vi "retrieveData.vi"(8 "error in (no error)":errorcluster, 11 "TemperatureSensor in":refnum<class "TemperatureSensor.lvclass">) -> (0 "error out":errorcluster, 2 "Temperature Measured":dbl[unit], 3 "TemperatureSensor out":refnum<class "TemperatureSensor.lvclass">)   [LabVIEW 2013, in "TemperatureSensor.lvclass"]
uses:
  TemperatureSensor.lvclass
  TemperatureSensor.lvclass/TemperatureSensor.ctl
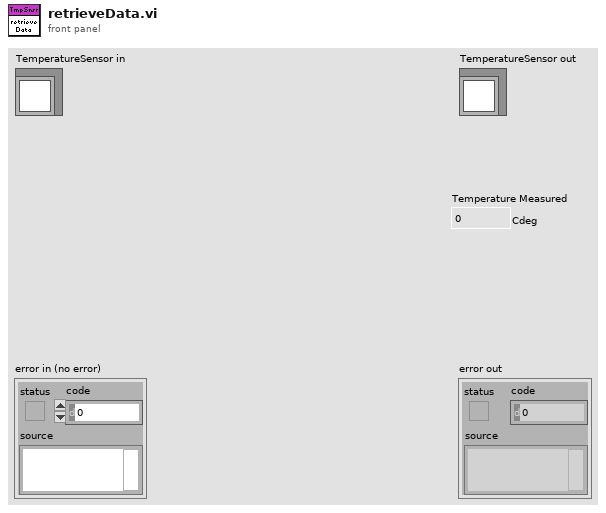
[diagram p1: front panel]
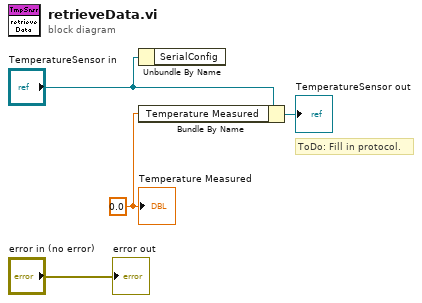
[diagram p0: block diagram]
diagram:
  w1 = dbl[unit] 0.0 ("Temperature Measured")
  # "ToDo: Fill in protocol."
  n1 = Unbundle By Name("TemperatureSensor in") -> ()  [unwired: 1 out]
  n2 = Bundle By Name(cluster="TemperatureSensor in", "Temperature Measured"=w1) -> (→"TemperatureSensor out":refnum<class "TemperatureSensor.lvclass">)
  "error out" <- "error in (no error)"
  "Temperature Measured" <- w1
